vi "Data_Process_Spectrum.vi"(7 "wfm info":T1, 8 "error in":errorcluster, 11 "dataset":i16[](array[numeric])) -> (0 "error out":errorcluster caption="sortie d'erreur", 2 "Frequency Spectrum":cluster{sgl[], sgl[]}, 3 "Dataset Signal":cluster{sgl[], sgl[]})   [LabVIEW 2017]
uses:
  Global_Variables.vi
  <vilib>/Analysis/NI_AALPro.lvlib
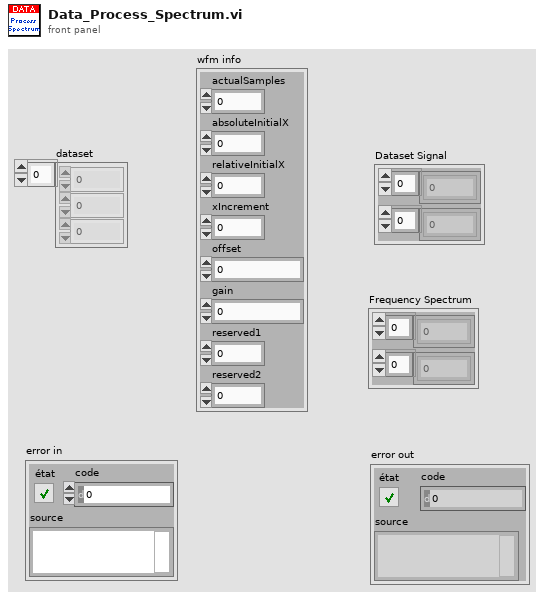
[diagram p1: front panel]
types:
  T1 = cluster{"actualSamples":i32, "absoluteInitialX":dbl, "relativeInitialX":dbl, "xIncrement":dbl, "offset":dbl, "gain":dbl, "reserved1":dbl, "reserved2":dbl}
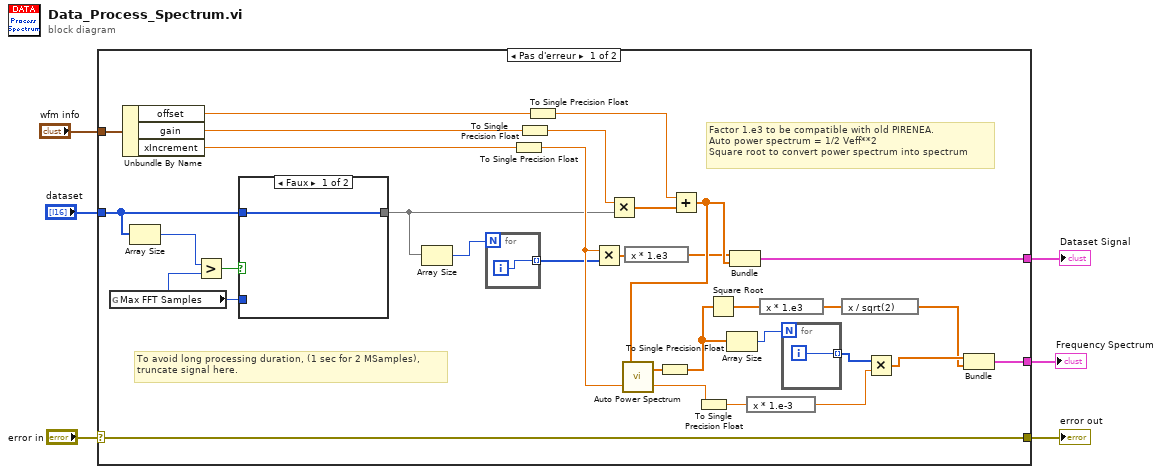
[diagram p0: block diagram]
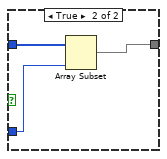
[diagram p2: hidden frame]
diagram:
  n1 = case shown="Pas d'erreur" "error in" {
    selector: "error in" -> [w36 w45]
    tunnel: [w38 _] -> w3
    tunnel: "dataset" -> [w9 _]
    tunnel: [w36 w45] -> w4
    tunnel: [w30 _] -> w1
    tunnel: "wfm info" -> [w28 _]
    frame No Error {
      # "To avoid long processing duration, (1 sec for 2 MSamples),\ntruncate signal here."
      # "Factor 1.e3 to be compatible with old PIRENEA.\nAuto power spectrum = 1/2 Veff**2\nSquare root to convert power spectrum into spectrum"
      n2 = global read "Global_Variables.vi" "Max FFT Samples"() -> (w7:i32)
      n3 = Unbundle By Name(w28) -> ("offset"=w27:dbl, "gain"=w26:dbl, "xIncrement"=w25:dbl)
      n4 = Array Size(array=w9) -> (size(s)=w8:i32)
      n5 = Greater?(x=w8, y=w7) -> (0:w11:bool)
      n6 = case shown="Faux" w11 {
        tunnel: w9 -> [w39 w42]
        tunnel: [w39 w41] -> w10
        tunnel: w7 -> [_ w40]
        frame False {
        }
        frame True {
          n7 = Array Subset(array=w42, length=w40) -> (w41:i16[])  [unwired: 1 in]
        }
      }
      n8 = Array Size(array=w10) -> (size(s)=w12:i32)
      n9 = for {
        N: w12 -> [_]
        tunnel: [w43] -> w15 mode=indexing
        i -> [w43]
      }
      n10 = To Single Precision Float(number=w25) -> (single precision float=w22:sgl)
      n11 = To Single Precision Float(number=w26) -> (single precision float=w23:sgl)
      n12 = To Single Precision Float(number=w27) -> (single precision float=w24:sgl)
      n13 = Multiply(x=w22, y=w15) -> (x*y=w14:sgl[])
      n14 = Multiply(x=w23, y=w10) -> (x*y=w37:sgl[])
      n15 = expression code="x * 1.e3"(w14) -> (w13:sgl[])
      n16 = Add(x=w24, y=w37) -> (x+y=w31:sgl[])
      n17 = call <vilib>:"Auto Power Spectrum.vi"("dt"=w22, "Signal (V)"=w31) -> ("df"=w33:dbl, "Power Spectrum (V^2 rms)"=w29:dbl[])
      n18 = To Single Precision Float(number=w29) -> (single precision float=w18:sgl[])
      n19 = To Single Precision Float(number=w33) -> (single precision float=w17:sgl)
      n20 = Square Root(x=w18) -> (sqrt(x)=w20:sgl[])
      n21 = Array Size(array=w18) -> (size(s)=w35:i32)
      n22 = Bundle(w13, w31) -> (w38:cluster{sgl[], sgl[]})  [unwired: 1 in]
      n23 = expression code="x * 1.e-3"(w17) -> (w32:sgl)
      n24 = expression code="x * 1.e3"(w20) -> (w19:sgl[])
      n25 = for {
        N: w35 -> [_]
        tunnel: [w44] -> w34 mode=indexing
        i -> [w44]
      }
      n26 = expression code="x / sqrt(2)"(w19) -> (w16:sgl[])
      n27 = Multiply(x=w34, y=w32) -> (x*y=w21:sgl[])
      n28 = Bundle(w21, w16) -> (w30:cluster{sgl[], sgl[]})  [unwired: 1 in]
    }
    frame Error {
    }
  }
  "Dataset Signal" <- w3
  "error out" <- w4
  "Frequency Spectrum" <- w1
